vi "Record_Snapshot.vi"(8 "error in (no error)":errorcluster, 10 "Data In":T4 {"Frame Data"."Image Type" items=["Grayscale (U8)", "Grayscale (I16)", "Grayscale (SGL)", "Complex (CSG)", "RGB (U32)", "HSL (U32)", "RGB (U64)", "Grayscale (U16)"]}, 11 "Recording Data":T1) -> (0 "error out":errorcluster, 3 "Recording Data Out":T1)   [LabVIEW 2017, in "ImageAcquisitionLibrary.lvlib"]
uses:
  ImageAcquisitionLibrary.lvlib
  Acquisition/AcquireData.ctl
  RecordingData.ctl
  <vilib>/vision/Image Controls.llb/IMAQ Image.ctl
  <vilib>/vision/Avi.llb/IMAQ AVI2 Refnum.ctl
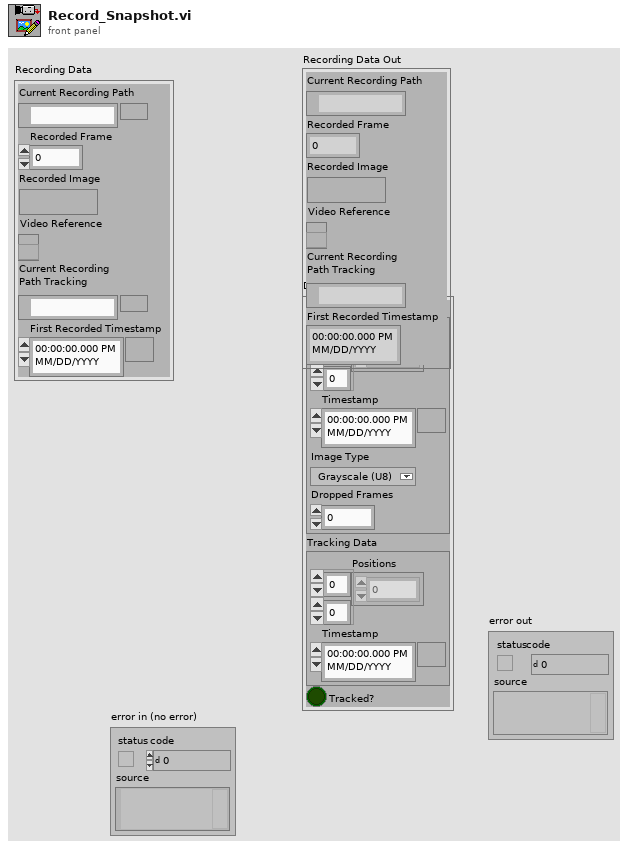
[diagram p1: front panel]
types:
  T1 = typedef "ImageAcquisitionLibrary.lvlib/RecordingData.ctl" = cluster{"Current Recording Path":path, "Recorded Frame":i32, "Recorded Image":T2, "Video Reference":T3, "Current Recording \nPath Tracking":path, "First Recorded Timestamp":timestamp}
  T2 = typedef "IMAQ Image.ctl" = refnum<image>
  T3 = typedef "IMAQ AVI2 Refnum.ctl" = refnum<k20>
  T4 = typedef "ImageAcquisitionLibrary.lvlib/AcquireData.ctl" = cluster{"Frame Data":cluster{"Image":u32[][], "Timestamp":timestamp, "Image Type":T5, "Dropped Frames":u32}, "Tracking Data":cluster{"Positions":dbl[][], "Timestamp":timestamp}, "Tracked?":bool}
  T5 = typedef "Image Type" = u32
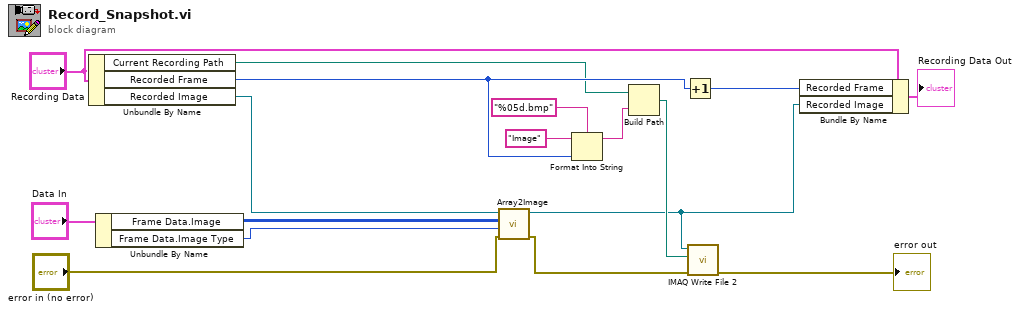
[diagram p0: block diagram]
diagram:
  n1 = Unbundle By Name("Recording Data") -> ("Current Recording Path"=w10:path, "Recorded Frame"=w11:i32, "Recorded Image"=w5:T2)
  n2 = Unbundle By Name("Data In") -> ("Frame Data.Image"=w4:u32[][], "Frame Data.Image Type"=w6:T5)
  n3 = call "Array2Image.vi"("error in (no error)"="error in (no error)", "Image Type"=w6, "Image Pixels (U32)"=w4, "Image 2"=w5) -> ("error out"=w2:errorcluster, "Image"=w1:T2)  [unwired: 6 in]
  n4 = Format Into String(format string="%05d.bmp", initial string="Image" ("input 1"), w11) -> (resulting string=w16:string)  [unwired: 1 in, 1 out]
  n5 = Build Path(base path=w10, name or relative path=w16) -> (appended path=w14:path)
  n6 = Increment(x=w11) -> (x+1=w8:i32)
  n7 = call-poly "IMAQ Write File 2"("error in (no error)"=w2, "File Path"=w14, "Image"=w1) -> ("error out"=→"error out":errorcluster)  [unwired: 7 in, 1 out]
  n8 = Bundle By Name(cluster="Recording Data", "Recorded Frame"=w8, "Recorded Image"=w1) -> (→"Recording Data Out":T1)
